vi "Command RPORT.vi"(0 "Serial Devices in":refnum<class "Serial Devices.lvclass">, 1 "Device":string, 7 "Port":u8, 11 "error in (no error)":errorcluster) -> (4 "Serial Devices out":refnum<class "Serial Devices.lvclass">, 6 "Command":string, 10 "Expected":string, 15 "error out":errorcluster)   [LabVIEW 2019, in "Serial Devices.lvlib" / "Serial Devices.lvclass"]
uses:
  Serial Devices.lvclass
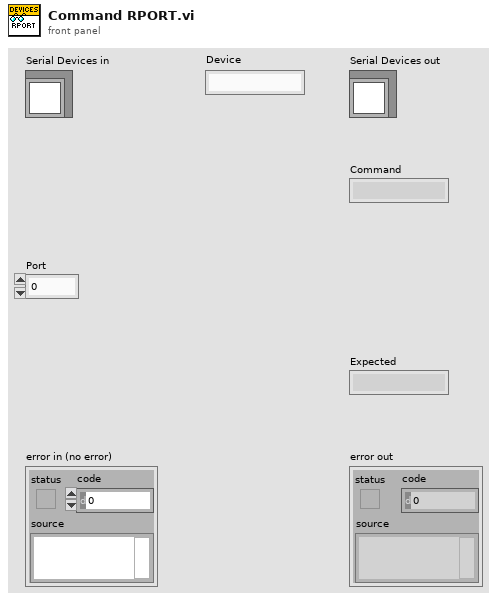
[diagram p1: front panel]
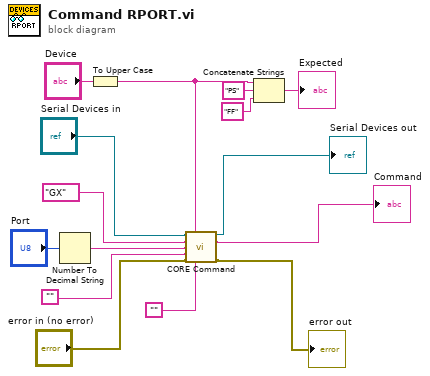
[diagram p0: block diagram]
diagram:
  n1 = Number To Decimal String(number="Port") -> (decimal integer string=w8:string)  [unwired: 1 in]
  n2 = To Upper Case(1:"Device") -> (0:w4:string)
  n3 = call "CORE Command.vi"("Serial Devices in"="Serial Devices in", "Device"=w4, "Command"="GX", "Chanel-Puerto"=w8, "Param-Pin"="", "error in (no error)"="error in (no error)", "Valor"="") -> ("Serial Devices out"=→"Serial Devices out":refnum<class "Serial Devices.lvclass">, "Command"=→"Command":string, "error out"=→"error out":errorcluster)  [unwired: 5 in, 1 out]
  n4 = Concatenate Strings(w4, "PS" ("string"), "FF" ("string")) -> (→"Expected":string)
